vi "pharosClose.vi"   [LabVIEW 2017]
uses:
  globalDevices.vi
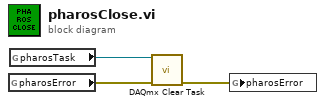
[diagram p0: block diagram]
diagram:
  n1 = global read "globalDevices.vi" "pharosError"() -> (w3:errorcluster)
  n2 = global read "globalDevices.vi" "pharosTask"() -> (w2:refnum<k21>)
  n3 = call <vilib>:"DAQmx Clear Task.vi"("task in"=w2, "error in"=w3) -> ("error out"=w1:errorcluster)  [unwired: 13 in]
  n4 = global write "globalDevices.vi" "pharosError"(w1) -> ()
